vi "V-Meter Shutdown (2000).vi"(8 "error in (no error)":errorcluster, 11 "VISA resource name in":refnum<visa-resource-name>) -> (0 "error out":errorcluster, 3 "VISA resource name out":refnum<visa-resource-name>)   [LabVIEW 2016, in "Hall Effect Library.lvlib"]
uses:
  Hall Effect Library.lvlib
  <instrlib>/Keithley 2000/Keithley 2000.lvlib
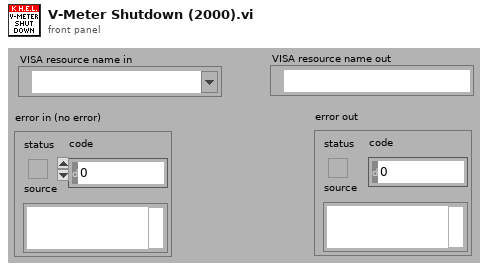
[diagram p1: front panel]
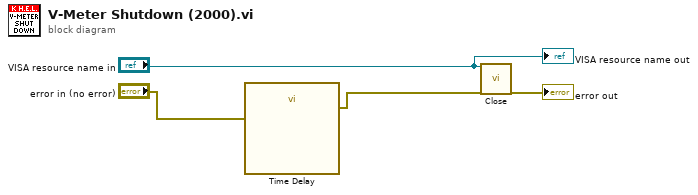
[diagram p0: block diagram]
diagram:
  n1 = call "Time Delay"("error in (no error)"="error in (no error)") -> ("error out"=w1:errorcluster)  [unwired: 10 in]
  n2 = call <instrlib>:"Close.vi"("VISA resource name"="VISA resource name in", "error in (no error)"=w1) -> ("error out"=→"error out":errorcluster)  [unwired: 17 out]
  "VISA resource name out" <- "VISA resource name in"
